vi "Hardware-DiffIO-Host.vi"() -> ()   [LabVIEW 2016]
uses:
  <vilib>/Powertrain Controls/Device Drivers/DCM/Diff IO/RT/Setup.ctl
  <vilib>/Powertrain Controls/Device Drivers/DCM/Diff IO/FPGA/Mode.ctl
  <vilib>/Powertrain Controls/Device Drivers/DCM/Diff IO/RT/Angle Control.ctl
  <vilib>/Powertrain Controls/Device Drivers/DCM/Diff IO/RT/Results.ctl
  Shared/Typedefs/DiffIO-PWM-Settings.ctl
  Shared/Typedefs/DiffIO-PWM-Settings-Array.ctl
  <vilib>/Powertrain Controls/Device Drivers/DCM/Diff IO/FPGA/DCM - FPGA - Diff IO.lvlib
  Shared/DSI-Shared.lvlib
  <vilib>/Powertrain Controls/Device Drivers/DCM/Diff IO/RT/DCM - RT - Diff IO.lvlib
panel:
  in  "_Hidden":enum32{"Page 1"}(tab)
  in  "Setup":T1[](array[typedef])=[{"Mode"=enum."Off", "Capture Start [DBTDC]"=0.0, "Capture End [DBTDC]"=0.0, "Polarity"=FALSE, "Frequency [Hz]"=0.0, "Duty Cycle [%]"=0.0, "TDC Offset [CAD]"=0.0, "Window Start [DBTDC]"=0.0, "Window End [DBTDC]"=0.0, "Angles"=[{"Enable"=FALSE, "Location [DBTDC]"=0.0, "Duration [s]"=0.0}, {"Enable"=FALSE, "Location [DBTDC]"=0.0, "Duration [s]"=0.0}, {"Enable"=FALSE, "Location [DBTDC]"=0.0, "Duration [s]"=0.0}, {"Enable"=FALSE, "Location [DBTDC]"=0.0, "Duration [s]"=0.0}], "Skip Fire"=FALSE, "Skip Fire Index"=0}, {"Mode"=enum."Off", "Capture Start [DBTDC]"=0.0, "Capture End [DBTDC]"=0.0, "Polarity"=FALSE, "Frequency [Hz]"=0.0, "Duty Cycle [%]"=0.0, "TDC Offset [CAD]"=0.0, "Window Start [DBTDC]"=0.0, "Window End [DBTDC]"=0.0, "Angles"=[{"Enable"=FALSE, "Location [DBTDC]"=0.0, "Duration [s]"=0.0}, {"Enable"=FALSE, "Location [DBTDC]"=0.0, "Duration [s]"=0.0}, {"Enable"=FALSE, "Location [DBTDC]"=0.0, "Duration [s]"=0.0}, {"Enable"=FALSE, "Location [DBTDC]"=0.0, "Duration [s]"=0.0}], "Skip Fire"=FALSE, "Skip Fire Index"=0}, {"Mode"=enum."Off", "Capture Start [DBTDC]"=0.0, "Capture End [DBTDC]"=0.0, "Polarity"=FALSE, "Frequency [Hz]"=0.0, "Duty Cycle [%]"=0.0, "TDC Offset [CAD]"=0.0, "Window Start [DBTDC]"=0.0, "Window End [DBTDC]"=0.0, "Angles"=[{"Enable"=FALSE, "Location [DBTDC]"=0.0, "Duration [s]"=0.0}, {"Enable"=FALSE, "Location [DBTDC]"=0.0, "Duration [s]"=0.0}, {"Enable"=FALSE, "Location [DBTDC]"=0.0, "Duration [s]"=0.0}, {"Enable"=FALSE, "Location [DBTDC]"=0.0, "Duration [s]"=0.0}], "Skip Fire"=FALSE, "Skip Fire Index"=0}, {"Mode"=enum."Off", "Capture Start [DBTDC]"=0.0, "Capture End [DBTDC]"=0.0, "Polarity"=FALSE, "Frequency [Hz]"=0.0, "Duty Cycle [%]"=0.0, "TDC Offset [CAD]"=0.0, "Window Start [DBTDC]"=0.0, "Window End [DBTDC]"=0.0, "Angles"=[{"Enable"=FALSE, "Location [DBTDC]"=0.0, "Duration [s]"=0.0}, {"Enable"=FALSE, "Location [DBTDC]"=0.0, "Duration [s]"=0.0}, {"Enable"=FALSE, "Location [DBTDC]"=0.0, "Duration [s]"=0.0}, {"Enable"=FALSE, "Location [DBTDC]"=0.0, "Duration [s]"=0.0}], "Skip Fire"=FALSE, "Skip Fire Index"=0}, {"Mode"=enum."Off", "Capture Start [DBTDC]"=0.0, "Capture End [DBTDC]"=0.0, "Polarity"=FALSE, "Frequency [Hz]"=0.0, "Duty Cycle [%]"=0.0, "TDC Offset [CAD]"=0.0, "Window Start [DBTDC]"=0.0, "Window End [DBTDC]"=0.0, "Angles"=[{"Enable"=FALSE, "Location [DBTDC]"=0.0, "Duration [s]"=0.0}, {"Enable"=FALSE, "Location [DBTDC]"=0.0, "Duration [s]"=0.0}, {"Enable"=FALSE, "Location [DBTDC]"=0.0, "Duration [s]"=0.0}, {"Enable"=FALSE, "Location [DBTDC]"=0.0, "Duration [s]"=0.0}], "Skip Fire"=FALSE, "Skip Fire Index"=0}, {"Mode"=enum."Off", "Capture Start [DBTDC]"=0.0, "Capture End [DBTDC]"=0.0, "Polarity"=FALSE, "Frequency [Hz]"=0.0, "Duty Cycle [%]"=0.0, "TDC Offset [CAD]"=0.0, "Window Start [DBTDC]"=0.0, "Window End [DBTDC]"=0.0, "Angles"=[{"Enable"=FALSE, "Location [DBTDC]"=0.0, "Duration [s]"=0.0}, {"Enable"=FALSE, "Location [DBTDC]"=0.0, "Duration [s]"=0.0}, {"Enable"=FALSE, "Location [DBTDC]"=0.0, "Duration [s]"=0.0}, {"Enable"=FALSE, "Location [DBTDC]"=0.0, "Duration [s]"=0.0}], "Skip Fire"=FALSE, "Skip Fire Index"=0}, {"Mode"=enum."Off", "Capture Start [DBTDC]"=0.0, "Capture End [DBTDC]"=0.0, "Polarity"=FALSE, "Frequency [Hz]"=0.0, "Duty Cycle [%]"=0.0, "TDC Offset [CAD]"=0.0, "Window Start [DBTDC]"=0.0, "Window End [DBTDC]"=0.0, "Angles"=[{"Enable"=FALSE, "Location [DBTDC]"=0.0, "Duration [s]"=0.0}, {"Enable"=FALSE, "Location [DBTDC]"=0.0, "Duration [s]"=0.0}, {"Enable"=FALSE, "Location [DBTDC]"=0.0, "Duration [s]"=0.0}, {"Enable"=FALSE, "Location [DBTDC]"=0.0, "Duration [s]"=0.0}], "Skip Fire"=FALSE, "Skip Fire Index"=0}, {"Mode"=enum."Off", "Capture Start [DBTDC]"=0.0, "Capture End [DBTDC]"=0.0, "Polarity"=FALSE, "Frequency [Hz]"=0.0, "Duty Cycle [%]"=0.0, "TDC Offset [CAD]"=0.0, "Window Start [DBTDC]"=0.0, "Window End [DBTDC]"=0.0, "Angles"=[{"Enable"=FALSE, "Location [DBTDC]"=0.0, "Duration [s]"=0.0}, {"Enable"=FALSE, "Location [DBTDC]"=0.0, "Duration [s]"=0.0}, {"Enable"=FALSE, "Location [DBTDC]"=0.0, "Duration [s]"=0.0}, {"Enable"=FALSE, "Location [DBTDC]"=0.0, "Duration [s]"=0.0}], "Skip Fire"=FALSE, "Skip Fire Index"=0}] {"Skip Fire Index" max=7; "Angles"."Duration [s]" format="%#_3p"; "Frequency [Hz]" format="%#_3p"}
  in  "_Refresh":bool
  in  "AdaptMode":u32
  in  "ChannelNames":string
  out "State":u8
  out "Results":T4[](array[typedef]) {"Duty Cycle [%]" format="%#_3g"; "Frequency [Hz]" format="%#_3p"}
  in  "PWMSettings":T5=[{"PWM-TimingMode"=enum."Frequency", "PWM-Frequency"=0.0, "PWM-Period"=0.0, "PWM-ControlMode"=enum."Duty Cycle", "PWM-DutyCycle"=0.0, "PWM-PulseWidth"=0.0}, {"PWM-TimingMode"=enum."Frequency", "PWM-Frequency"=0.0, "PWM-Period"=0.0, "PWM-ControlMode"=enum."Duty Cycle", "PWM-DutyCycle"=0.0, "PWM-PulseWidth"=0.0}, {"PWM-TimingMode"=enum."Frequency", "PWM-Frequency"=0.0, "PWM-Period"=0.0, "PWM-ControlMode"=enum."Duty Cycle", "PWM-DutyCycle"=0.0, "PWM-PulseWidth"=0.0}, {"PWM-TimingMode"=enum."Frequency", "PWM-Frequency"=0.0, "PWM-Period"=0.0, "PWM-ControlMode"=enum."Duty Cycle", "PWM-DutyCycle"=0.0, "PWM-PulseWidth"=0.0}, {"PWM-TimingMode"=enum."Frequency", "PWM-Frequency"=0.0, "PWM-Period"=0.0, "PWM-ControlMode"=enum."Duty Cycle", "PWM-DutyCycle"=0.0, "PWM-PulseWidth"=0.0}, {"PWM-TimingMode"=enum."Frequency", "PWM-Frequency"=0.0, "PWM-Period"=0.0, "PWM-ControlMode"=enum."Duty Cycle", "PWM-DutyCycle"=0.0, "PWM-PulseWidth"=0.0}, {"PWM-TimingMode"=enum."Frequency", "PWM-Frequency"=0.0, "PWM-Period"=0.0, "PWM-ControlMode"=enum."Duty Cycle", "PWM-DutyCycle"=0.0, "PWM-PulseWidth"=0.0}, {"PWM-TimingMode"=enum."Frequency", "PWM-Frequency"=0.0, "PWM-Period"=0.0, "PWM-ControlMode"=enum."Duty Cycle", "PWM-DutyCycle"=0.0, "PWM-PulseWidth"=0.0}] caption="Advanced PWM Settings" {"PWM-Period" format="%#_2p"; "PWM-PulseWidth" format="%#_2p"; "PWM-DutyCycle" format="%#_2p"; "PWM-Frequency" format="%#_2p"}
  in  "Filters":sgl[](array[numeric]) caption="Digital Filter" format="%#.2p"
  in  "_Filter":sgl caption="Digital Filter [s]" format="%#_4p"
  in  "_PWM Settings Element":T6 caption="Advanced PWM Settings" {"PWM-Period" format="%#_2p"; "PWM-PulseWidth" format="%#_2p"; "PWM-DutyCycle" format="%#_2p"; "PWM-Frequency" format="%#_2p"}
  in  "_Setup Tab":enum32{"Page 1"}(tab)
  out "_ResultsElement":T4 caption="Channel Results" {"Duty Cycle [%]" format="%#_3g"; "Frequency [Hz]" format="%#_3p"}
  in  "_SetupElement":T1={"Mode"=enum."Off", "Capture Start [DBTDC]"=0.0, "Capture End [DBTDC]"=0.0, "Polarity"=FALSE, "Frequency [Hz]"=0.0, "Duty Cycle [%]"=0.0, "TDC Offset [CAD]"=0.0, "Window Start [DBTDC]"=0.0, "Window End [DBTDC]"=0.0, "Angles"=[{"Enable"=FALSE, "Location [DBTDC]"=0.0, "Duration [s]"=0.0}, {"Enable"=FALSE, "Location [DBTDC]"=0.0, "Duration [s]"=0.0}, {"Enable"=FALSE, "Location [DBTDC]"=0.0, "Duration [s]"=0.0}, {"Enable"=FALSE, "Location [DBTDC]"=0.0, "Duration [s]"=0.0}], "Skip Fire"=FALSE, "Skip Fire Index"=0} caption="Command Setup" {"Skip Fire Index" max=7; "Angles"."Duration [s]" format="%#_3p"; "Frequency [Hz]" format="%#_3p"}
  in  "_AdaptMode":bool caption="Adapt Mode"
  in  "_Channel Name":string caption="Name"
  in  "_DiffIO Channels":i32[](listbox) caption="Differential Digital I/O Channel Summary"
  # "Differential Digital I/O Setup & Control"
  # "Channel Settings"
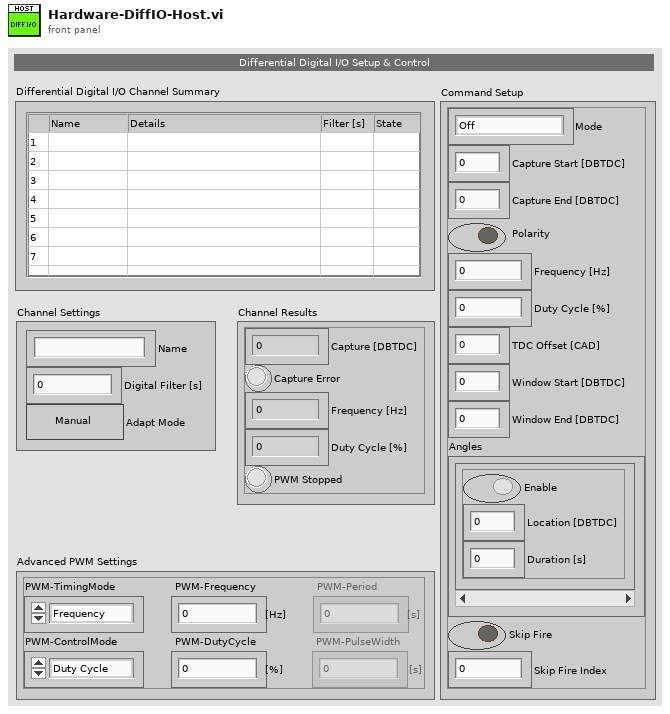
[diagram p1: front panel]
types:
  T1 = typedef "DCM - RT - Diff IO.lvlib/Setup.ctl" = cluster{"Mode":T2, "Capture Start [DBTDC]":sgl, "Capture End [DBTDC]":sgl, "Polarity":bool, "Frequency [Hz]":sgl, "Duty Cycle [%]":sgl, "TDC Offset [CAD]":sgl, "Window Start [DBTDC]":sgl, "Window End [DBTDC]":sgl, "Angles":T3[], "Skip Fire":bool, "Skip Fire Index":u8}
  T2 = typedef "DCM - FPGA - Diff IO.lvlib/Mode.ctl" = enum8{"Off", "Input", "Pulse Width Modulation", "Engine Position Tracking", "Serial Out 1", "Serial Out 2"}
  T3 = typedef "DCM - RT - Diff IO.lvlib/Angle Control.ctl" = cluster{"Enable":bool, "Location [DBTDC]":sgl, "Duration [s]":sgl}
  T4 = typedef "DCM - RT - Diff IO.lvlib/Results.ctl" = cluster{"Capture [DBTDC]":sgl, "Capture Error":bool, "Frequency [Hz]":sgl, "Duty Cycle [%]":sgl, "PWM Stopped":bool}
  T5 = typedef "DSI-Shared.lvlib/DiffIO-PWM-Settings-Array.ctl" = T6[]
  T6 = typedef "DSI-Shared.lvlib/DiffIO-PWM-Settings.ctl" = cluster{"PWM-TimingMode":enum32{"Frequency", "Period"}, "PWM-Frequency":sgl, "PWM-Period":sgl, "PWM-ControlMode":enum32{"Duty Cycle", "Pulsewidth"}, "PWM-DutyCycle":sgl, "PWM-PulseWidth":sgl}
  T7 = enum8{"Enabled", "Disabled", "Disabled and Grayed Out"}
  T8 = enum32{"Invalid", "Standard", "Closed", "Hidden", "Minimized", "Maximized"}
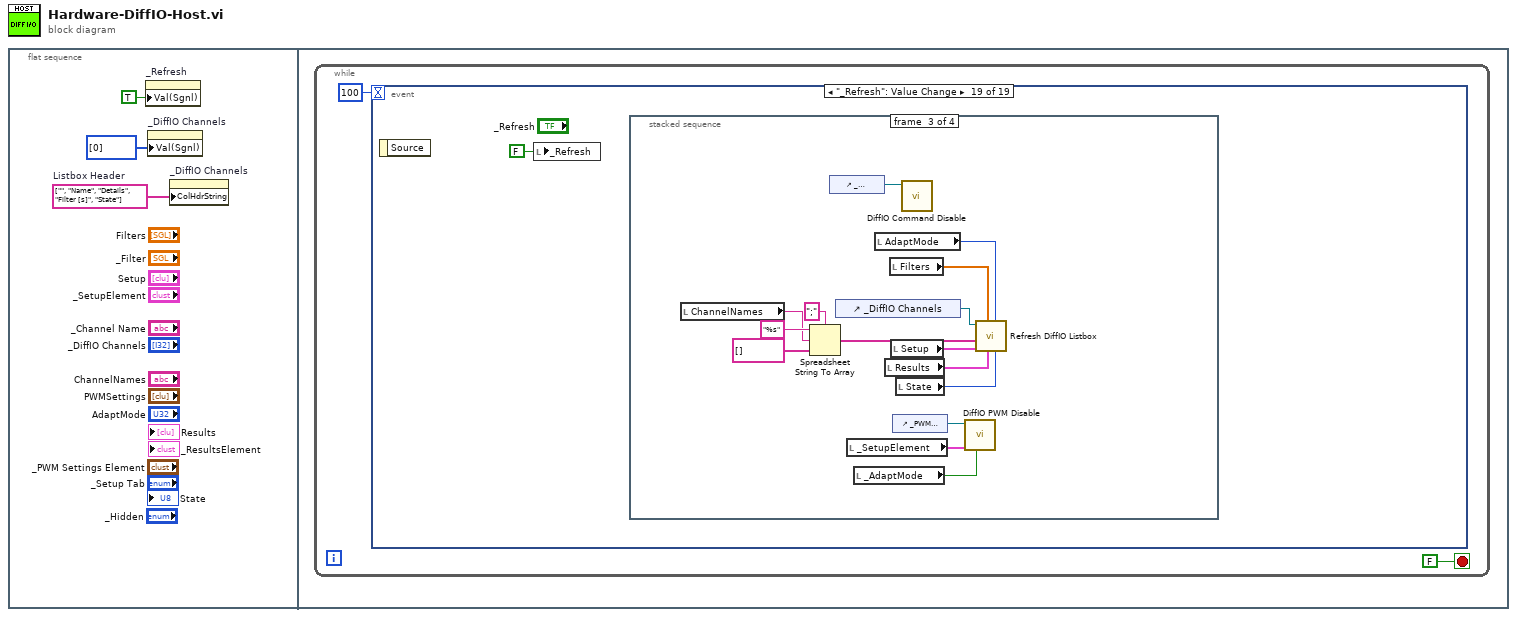
[diagram p0: block diagram]
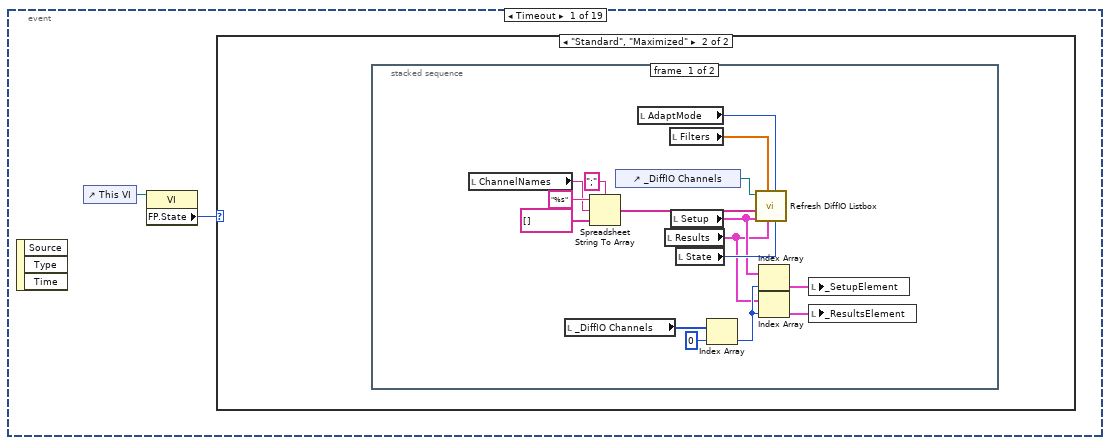
[diagram p2: hidden frame]
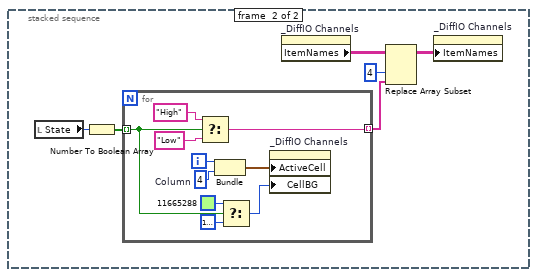
[diagram p4: hidden frame]
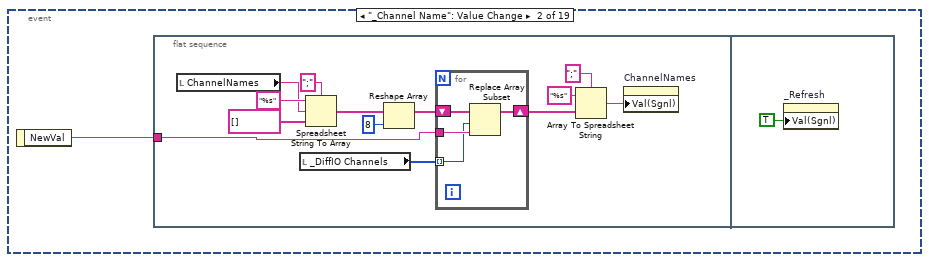
[diagram p5: hidden frame]
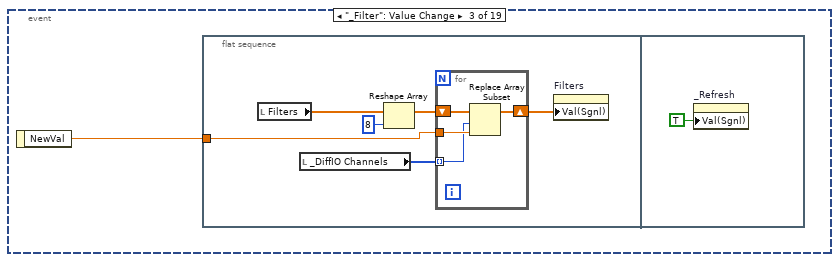
[diagram p6: hidden frame]
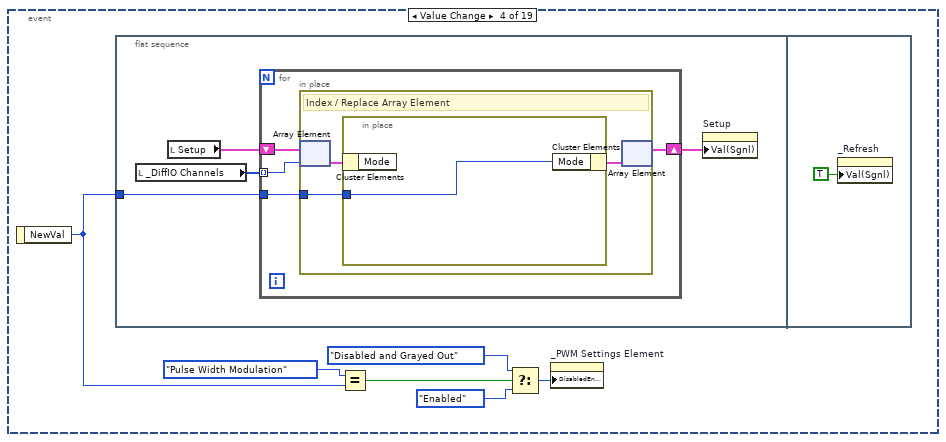
[diagram p7: hidden frame]
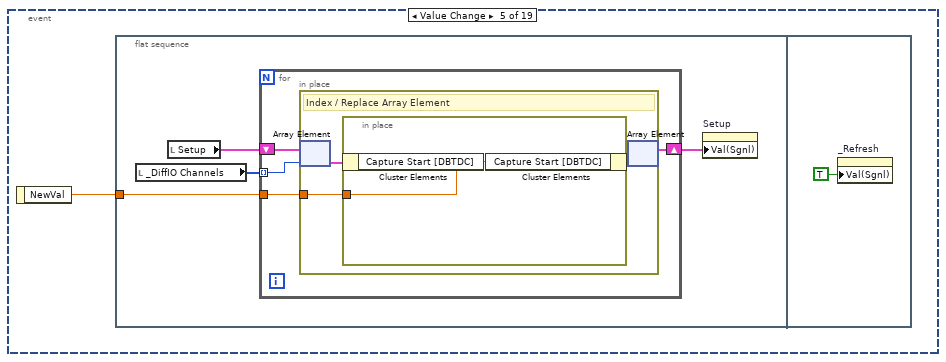
[diagram p8: hidden frame]
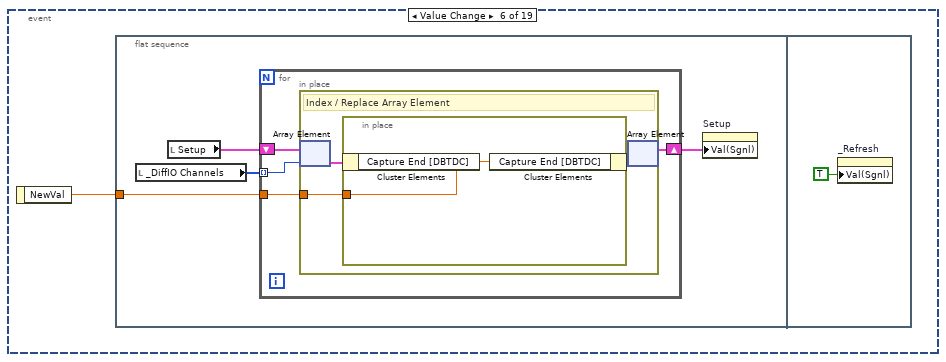
[diagram p9: hidden frame]
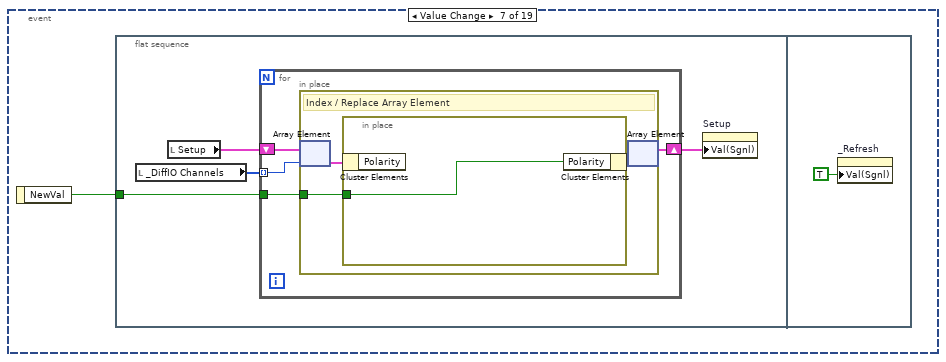
[diagram p10: hidden frame]
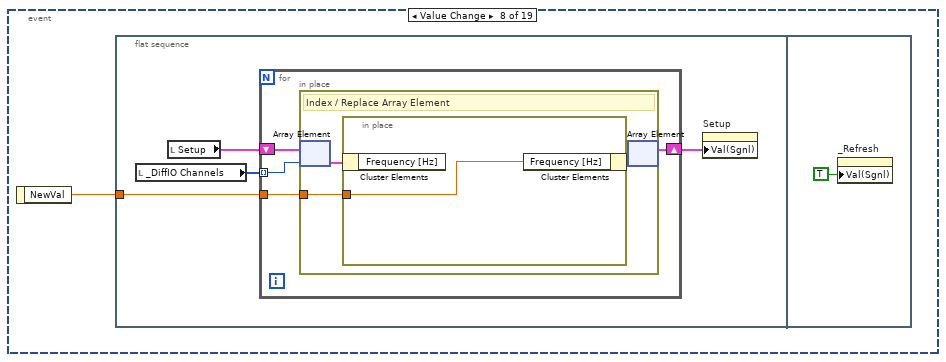
[diagram p11: hidden frame]
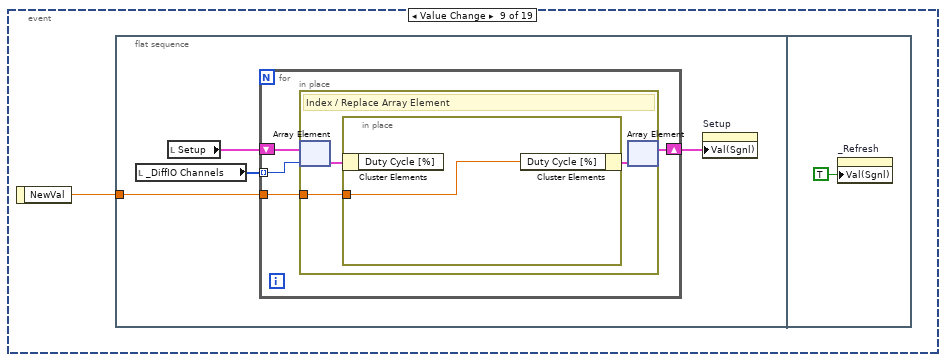
[diagram p12: hidden frame]
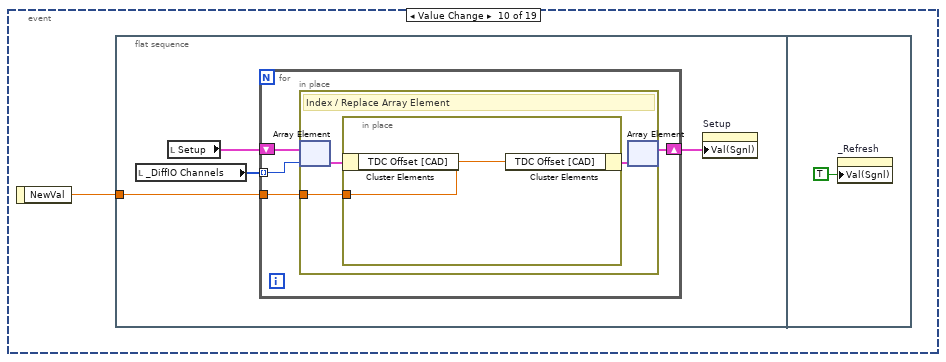
[diagram p13: hidden frame]
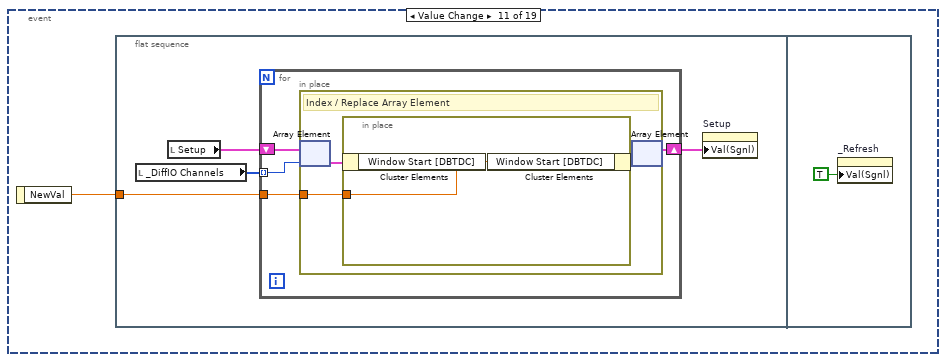
[diagram p14: hidden frame]
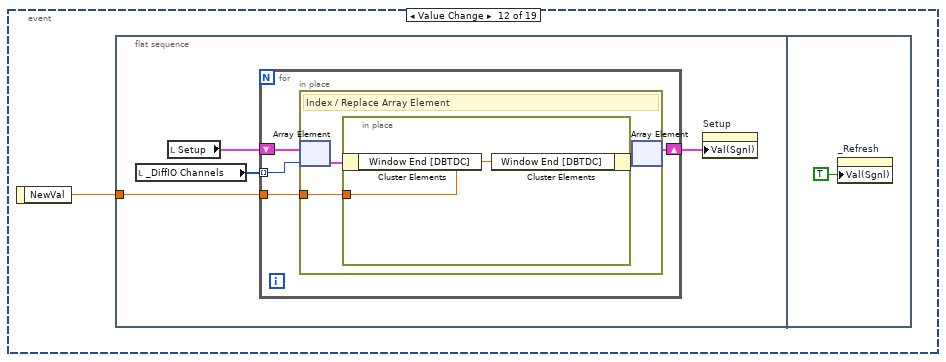
[diagram p15: hidden frame]
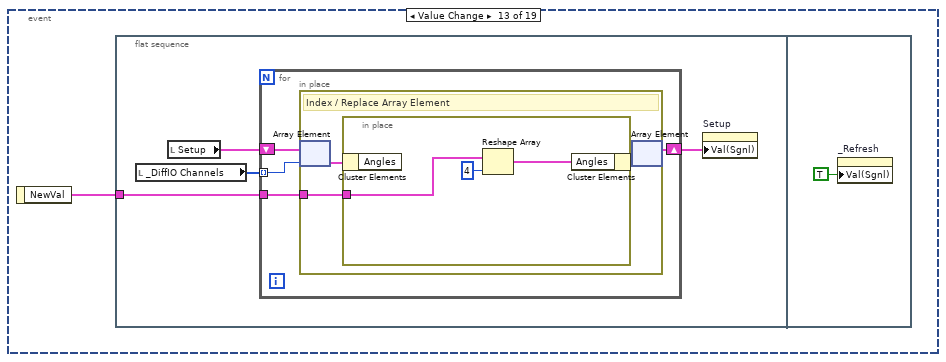
[diagram p16: hidden frame]
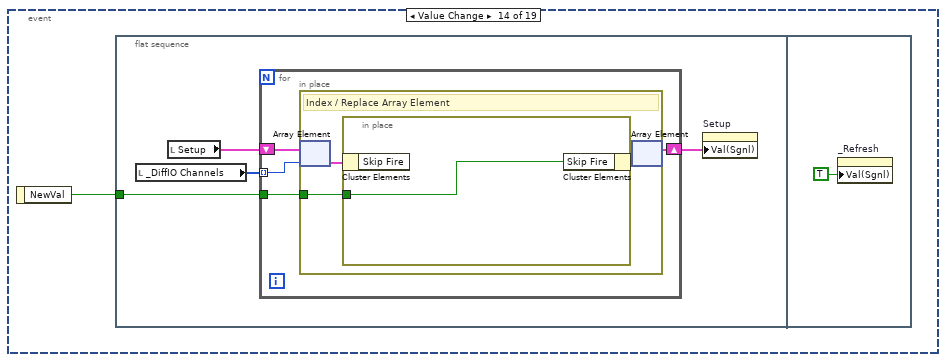
[diagram p17: hidden frame]
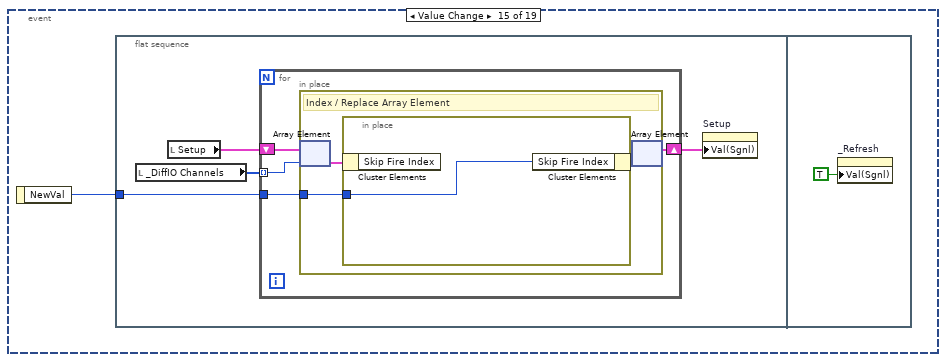
[diagram p18: hidden frame]
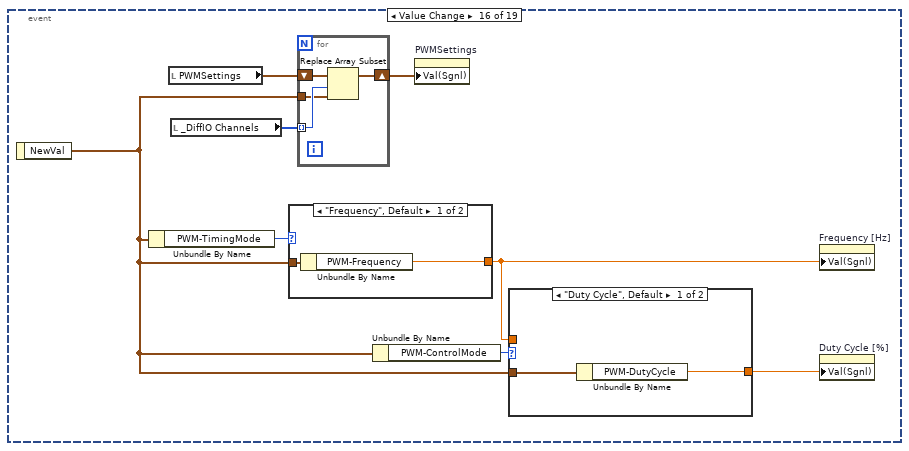
[diagram p19: hidden frame]
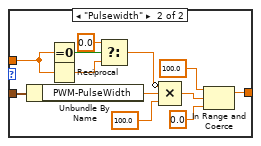
[diagram p20: hidden frame]
diagram:
  n1 = flat-sequence "Initialization code" {
    frame #0 {
      w3 = string[] ["", "Name", "Details", "Filter [s]", "State"]  # Listbox Header
      n2 = property on="_Refresh" class="Bool (strict)"("Val(Sgnl)"=TRUE ("Value (Signaling)")) -> ()  [unwired: 2 in, 2 out]
      n3 = property on="_DiffIO Channels" class="MCListbox (strict)"("Val(Sgnl)"=i32[] [0] ("Value (Signaling)")) -> ()  [unwired: 2 in, 2 out]
      n4 = property on="_DiffIO Channels" class="MCListbox (strict)"("ColHdrString"=w3) -> ()  [unwired: 2 in, 2 out]
    }
    frame #1 {
      n5 = while {
        stop <- FALSE stop-if-true
        n6 = event shown="[18] \"_Refresh\": Value Change" {
          selector: _ -> [_ _ _ _ _ _ _ _ _ _ _ _ _ _ _ _ _ _ _]
          dyn-events: _ -> [_ _ _ _ _ _ _ _ _ _ _ _ _ _ _ _ _ _ _]
          timeout: 100 -> [_ _ _ _ _ _ _ _ _ _ _ _ _ _ _ _ _ _ _]
          event Timeout {
            n7 = event-data() -> ()  [unwired: 4 out]
            n8 = control-ref of="This VI"() -> (w7:refnum<vi>)
            n9 = property class="VI"(reference=w7) -> ("FP.State"=w6:T8)  [unwired: 1 in, 2 out]
            n10 = case shown="\"Standard\", \"Maximized\"" w6 {
              frame "Invalid", Default {
              }
              frame "Standard", "Maximized" {
                n11 = stacked-sequence {
                  frame #0 {
                    n12 = local read "ChannelNames"() -> (w17:string)
                    n13 = local read "_DiffIO Channels"() -> (w22:i32[])
                    n14 = Spreadsheet String To Array(delimiter (Tab)=";", format string="%s", spreadsheet string=w17, array type (2D Dbl)=string[] []) -> (array=w16:string[])
                    n15 = control-ref of="_DiffIO Channels"() -> (w13:refnum<vi>)
                    n16 = local read "AdaptMode"() -> (w23:u32)
                    n17 = local read "Results"() -> (w8:T4[])
                    n18 = local read "Filters"() -> (w12:sgl[])
                    n19 = local read "Setup"() -> (w9:T1[])
                    n20 = local read "State"() -> (w14:u8)
                    n21 = Index Array(array=w22, index=0) -> (element=w10:i32)
                    n22 = call "Refresh DiffIO Listbox.vi"("_DiffIOState"=w14, "AdaptMode"=w23, "Results"=w8, "DigitalFilter"=w12, "Command"=w9, "Names"=w16, "_DiffIO Channels"=w13) -> ()  [unwired: 5 in]
                    n23 = Index Array(array=w9, index=w10) -> (element=w11:T1)
                    n24 = Index Array(array=w8, index=w10) -> (element=w20:T4)
                    n25 = local write "_SetupElement"(w11) -> ()
                    n26 = local write "_ResultsElement"(w20) -> ()
                  }
                  frame #1 {
                    n27 = local read "State"() -> (w27:u8)
                    n28 = Number To Boolean Array(number=w27) -> (Boolean array=w28:bool[])
                    n29 = for {
                      tunnel: w28 -> [w31] mode=indexing
                      tunnel: [w30] -> w25 mode=indexing
                      i -> [w38]
                      w39 = 4  # Column
                      n30 = Select(t="High" ("format string"), s=w31, f="Low" ("format string")) -> (s? t:f=w30:string)
                      n31 = Bundle(w38, "Column"=w39) -> (w37:cluster{i32, "Column":i32})  [unwired: 1 in]
                      n32 = Select(t=u32 11665288, s=w31, f=u32 16777226) -> (s? t:f=w34:u32)
                      n33 = property on="_DiffIO Channels" class="MCListbox (strict)"("ActiveCell"=w37, "CellBG"=w34) -> ()  [unwired: 2 in, 2 out]
                    }
                    n34 = property on="_DiffIO Channels" class="MCListbox (strict)"() -> ("ItemNames"=w26:string[][])  [unwired: 2 in, 2 out]
                    n35 = Replace Array Subset(array=w26, new element=w25, index (col)=4 ("disabled index (col)")) -> (w24:string[][])  [unwired: 1 in]
                    n36 = property on="_DiffIO Channels" class="MCListbox (strict)"("ItemNames"=w24) -> ()  [unwired: 2 in, 2 out]
                  }
                }
              }
            }
          }
          event "_Channel Name": Value Change {
            n37 = event-data() -> ("NewVal"=w40:string)  [unwired: 1 out]
            n38 = flat-sequence {
              tunnel: w40 -> [w42]
              frame #0 {
                n39 = local read "ChannelNames"() -> (w51:string)
                n40 = local read "_DiffIO Channels"() -> (w41:i32[])
                n41 = Spreadsheet String To Array(delimiter (Tab)=";", format string="%s", spreadsheet string=w51, array type (2D Dbl)=string[] []) -> (array=w49:string[])
                n42 = Reshape Array(w49, 8 ("dimension size")) -> (w44:string[])
                n43 = for {
                  tunnel: w42 -> [w55]
                  shift-right: [w57] -> w48
                  shift-left: w44 -> [w56]
                  tunnel: w41 -> [w54] mode=indexing
                  n44 = Replace Array Subset(array=w56, new element=w55, index=w54) -> (w57:string[])
                }
                n45 = Array To Spreadsheet String(delimiter (Tab)=";", array=w48, 3:"%s" ("format string")) -> (spreadsheet string=w45:string)
                n46 = property on="ChannelNames" class="Str"("Val(Sgnl)"=w45) -> ()  [unwired: 2 in, 2 out]
              }
              frame #1 {
                n47 = property on="_Refresh" class="Bool (strict)"("Val(Sgnl)"=TRUE ("Value (Signaling)")) -> ()  [unwired: 2 in, 2 out]
              }
            }
          }
          event "_Filter": Value Change {
            n48 = event-data() -> ("NewVal"=w59:sgl)  [unwired: 1 out]
            n49 = flat-sequence {
              tunnel: w59 -> [w63]
              frame #0 {
                n50 = local read "Filters"() -> (w61:sgl[])
                n51 = local read "_DiffIO Channels"() -> (w62:i32[])
                n52 = Reshape Array(w61, 8 ("dimension size")) -> (w65:sgl[])
                n53 = for {
                  tunnel: w63 -> [w67]
                  shift-right: [w69] -> w60
                  shift-left: w65 -> [w68]
                  tunnel: w62 -> [w66] mode=indexing
                  n54 = Replace Array Subset(array=w68, new element=w67, index=w66) -> (w69:sgl[])
                }
                n55 = property on="Filters" class="Arr (strict)"("Val(Sgnl)"=w60) -> ()  [unwired: 2 in, 2 out]
              }
              frame #1 {
                n56 = property on="_Refresh" class="Bool (strict)"("Val(Sgnl)"=TRUE ("Value (Signaling)")) -> ()  [unwired: 2 in, 2 out]
              }
            }
          }
          event Value Change {
            n57 = event-data() -> ("NewVal"=w71:T2)  [unwired: 1 out]
            n58 = flat-sequence {
              tunnel: w71 -> [w79]
              frame #0 {
                n59 = local read "_DiffIO Channels"() -> (w80:i32[])
                n60 = local read "Setup"() -> (w78:T1[])
                n61 = for {
                  tunnel: w80 -> [w83] mode=indexing
                  shift-right: [w82] -> w77
                  shift-left: w78 -> [w84]
                  tunnel: w79 -> [w81]
                  n62 = in-place {
                    in-place-border: w81 -> [w85]
                    # "Index / Replace Array Element"
                    n63 = in-place-array #1(w84, w83) -> (w87:T1)
                    n64 = in-place {
                      in-place-border: w85 -> [w88]
                      n65 = in-place-cluster #2(w87) -> ()  [unwired: 1 out]
                      n66 = in-place-cluster #2("Mode"=w88) -> (w86:T1)
                    }
                    n67 = in-place-array #1(w86) -> (w82:T1[])  [unwired: 1 out]
                  }
                }
                n68 = property on="Setup" class="Arr (strict)"("Val(Sgnl)"=w77) -> ()  [unwired: 2 in, 2 out]
              }
              frame #1 {
                n69 = property on="_Refresh" class="Bool (strict)"("Val(Sgnl)"=TRUE ("Value (Signaling)")) -> ()  [unwired: 2 in, 2 out]
              }
            }
            n70 = Equal?(x=Mode."Pulse Width Modulation" ("Mode"), y=w71) -> (x = y?=w73:bool)
            n71 = Select(t=T7."Disabled and Grayed Out" ("Disabled"), s=w73, f=T7."Enabled" ("Disabled")) -> (s? t:f=w72:T7)
            n72 = property on="_PWM Settings Element" class="Clust (strict)"("DisabledEnum"=w72) -> ()  [unwired: 2 in, 2 out]
          }
          event Value Change {
            n73 = event-data() -> ("NewVal"=w90:sgl)  [unwired: 1 out]
            n74 = flat-sequence {
              tunnel: w90 -> [w93]
              frame #0 {
                n75 = local read "_DiffIO Channels"() -> (w94:i32[])
                n76 = local read "Setup"() -> (w92:T1[])
                n77 = for {
                  tunnel: w94 -> [w97] mode=indexing
                  shift-right: [w96] -> w91
                  shift-left: w92 -> [w98]
                  tunnel: w93 -> [w95]
                  n78 = in-place {
                    in-place-border: w95 -> [w99]
                    # "Index / Replace Array Element"
                    n79 = in-place-array #3(w98, w97) -> (w101:T1)
                    n80 = in-place {
                      in-place-border: w99 -> [w102]
                      n81 = in-place-cluster #4(w101) -> ()  [unwired: 1 out]
                      n82 = in-place-cluster #4("Capture Start [DBTDC]"=w102) -> (w100:T1)
                    }
                    n83 = in-place-array #3(w100) -> (w96:T1[])  [unwired: 1 out]
                  }
                }
                n84 = property on="Setup" class="Arr (strict)"("Val(Sgnl)"=w91) -> ()  [unwired: 2 in, 2 out]
              }
              frame #1 {
                n85 = property on="_Refresh" class="Bool (strict)"("Val(Sgnl)"=TRUE ("Value (Signaling)")) -> ()  [unwired: 2 in, 2 out]
              }
            }
          }
          event Value Change {
            n86 = event-data() -> ("NewVal"=w104:sgl)  [unwired: 1 out]
            n87 = flat-sequence {
              tunnel: w104 -> [w107]
              frame #0 {
                n88 = local read "_DiffIO Channels"() -> (w108:i32[])
                n89 = local read "Setup"() -> (w106:T1[])
                n90 = for {
                  tunnel: w108 -> [w111] mode=indexing
                  shift-right: [w110] -> w105
                  shift-left: w106 -> [w112]
                  tunnel: w107 -> [w109]
                  n91 = in-place {
                    in-place-border: w109 -> [w113]
                    # "Index / Replace Array Element"
                    n92 = in-place-array #5(w112, w111) -> (w115:T1)
                    n93 = in-place {
                      in-place-border: w113 -> [w116]
                      n94 = in-place-cluster #6(w115) -> ()  [unwired: 1 out]
                      n95 = in-place-cluster #6("Capture End [DBTDC]"=w116) -> (w114:T1)
                    }
                    n96 = in-place-array #5(w114) -> (w110:T1[])  [unwired: 1 out]
                  }
                }
                n97 = property on="Setup" class="Arr (strict)"("Val(Sgnl)"=w105) -> ()  [unwired: 2 in, 2 out]
              }
              frame #1 {
                n98 = property on="_Refresh" class="Bool (strict)"("Val(Sgnl)"=TRUE ("Value (Signaling)")) -> ()  [unwired: 2 in, 2 out]
              }
            }
          }
          event Value Change {
            n99 = event-data() -> ("NewVal"=w118:bool)  [unwired: 1 out]
            n100 = flat-sequence {
              tunnel: w118 -> [w121]
              frame #0 {
                n101 = local read "_DiffIO Channels"() -> (w122:i32[])
                n102 = local read "Setup"() -> (w120:T1[])
                n103 = for {
                  tunnel: w122 -> [w125] mode=indexing
                  shift-right: [w124] -> w119
                  shift-left: w120 -> [w126]
                  tunnel: w121 -> [w123]
                  n104 = in-place {
                    in-place-border: w123 -> [w127]
                    # "Index / Replace Array Element"
                    n105 = in-place-array #7(w126, w125) -> (w129:T1)
                    n106 = in-place {
                      in-place-border: w127 -> [w130]
                      n107 = in-place-cluster #8(w129) -> ()  [unwired: 1 out]
                      n108 = in-place-cluster #8("Polarity"=w130) -> (w128:T1)
                    }
                    n109 = in-place-array #7(w128) -> (w124:T1[])  [unwired: 1 out]
                  }
                }
                n110 = property on="Setup" class="Arr (strict)"("Val(Sgnl)"=w119) -> ()  [unwired: 2 in, 2 out]
              }
              frame #1 {
                n111 = property on="_Refresh" class="Bool (strict)"("Val(Sgnl)"=TRUE ("Value (Signaling)")) -> ()  [unwired: 2 in, 2 out]
              }
            }
          }
          event Value Change {
            n112 = event-data() -> ("NewVal"=w132:sgl)  [unwired: 1 out]
            n113 = flat-sequence {
              tunnel: w132 -> [w135]
              frame #0 {
                n114 = local read "_DiffIO Channels"() -> (w136:i32[])
                n115 = local read "Setup"() -> (w134:T1[])
                n116 = for {
                  tunnel: w136 -> [w139] mode=indexing
                  shift-right: [w138] -> w133
                  shift-left: w134 -> [w140]
                  tunnel: w135 -> [w137]
                  n117 = in-place {
                    in-place-border: w137 -> [w141]
                    # "Index / Replace Array Element"
                    n118 = in-place-array #9(w140, w139) -> (w143:T1)
                    n119 = in-place {
                      in-place-border: w141 -> [w144]
                      n120 = in-place-cluster #10(w143) -> ()  [unwired: 1 out]
                      n121 = in-place-cluster #10("Frequency [Hz]"=w144) -> (w142:T1)
                    }
                    n122 = in-place-array #9(w142) -> (w138:T1[])  [unwired: 1 out]
                  }
                }
                n123 = property on="Setup" class="Arr (strict)"("Val(Sgnl)"=w133) -> ()  [unwired: 2 in, 2 out]
              }
              frame #1 {
                n124 = property on="_Refresh" class="Bool (strict)"("Val(Sgnl)"=TRUE ("Value (Signaling)")) -> ()  [unwired: 2 in, 2 out]
              }
            }
          }
          event Value Change {
            n125 = event-data() -> ("NewVal"=w146:sgl)  [unwired: 1 out]
            n126 = flat-sequence {
              tunnel: w146 -> [w149]
              frame #0 {
                n127 = local read "_DiffIO Channels"() -> (w150:i32[])
                n128 = local read "Setup"() -> (w148:T1[])
                n129 = for {
                  tunnel: w150 -> [w153] mode=indexing
                  shift-right: [w152] -> w147
                  shift-left: w148 -> [w154]
                  tunnel: w149 -> [w151]
                  n130 = in-place {
                    in-place-border: w151 -> [w155]
                    # "Index / Replace Array Element"
                    n131 = in-place-array #11(w154, w153) -> (w157:T1)
                    n132 = in-place {
                      in-place-border: w155 -> [w158]
                      n133 = in-place-cluster #12(w157) -> ()  [unwired: 1 out]
                      n134 = in-place-cluster #12("Duty Cycle [%]"=w158) -> (w156:T1)
                    }
                    n135 = in-place-array #11(w156) -> (w152:T1[])  [unwired: 1 out]
                  }
                }
                n136 = property on="Setup" class="Arr (strict)"("Val(Sgnl)"=w147) -> ()  [unwired: 2 in, 2 out]
              }
              frame #1 {
                n137 = property on="_Refresh" class="Bool (strict)"("Val(Sgnl)"=TRUE ("Value (Signaling)")) -> ()  [unwired: 2 in, 2 out]
              }
            }
          }
          event Value Change {
            n138 = event-data() -> ("NewVal"=w160:sgl)  [unwired: 1 out]
            n139 = flat-sequence {
              tunnel: w160 -> [w163]
              frame #0 {
                n140 = local read "_DiffIO Channels"() -> (w164:i32[])
                n141 = local read "Setup"() -> (w162:T1[])
                n142 = for {
                  tunnel: w164 -> [w167] mode=indexing
                  shift-right: [w166] -> w161
                  shift-left: w162 -> [w168]
                  tunnel: w163 -> [w165]
                  n143 = in-place {
                    in-place-border: w165 -> [w169]
                    # "Index / Replace Array Element"
                    n144 = in-place-array #13(w168, w167) -> (w171:T1)
                    n145 = in-place {
                      in-place-border: w169 -> [w172]
                      n146 = in-place-cluster #14(w171) -> ()  [unwired: 1 out]
                      n147 = in-place-cluster #14("TDC Offset [CAD]"=w172) -> (w170:T1)
                    }
                    n148 = in-place-array #13(w170) -> (w166:T1[])  [unwired: 1 out]
                  }
                }
                n149 = property on="Setup" class="Arr (strict)"("Val(Sgnl)"=w161) -> ()  [unwired: 2 in, 2 out]
              }
              frame #1 {
                n150 = property on="_Refresh" class="Bool (strict)"("Val(Sgnl)"=TRUE ("Value (Signaling)")) -> ()  [unwired: 2 in, 2 out]
              }
            }
          }
          event Value Change {
            n151 = event-data() -> ("NewVal"=w174:sgl)  [unwired: 1 out]
            n152 = flat-sequence {
              tunnel: w174 -> [w177]
              frame #0 {
                n153 = local read "_DiffIO Channels"() -> (w178:i32[])
                n154 = local read "Setup"() -> (w176:T1[])
                n155 = for {
                  tunnel: w178 -> [w181] mode=indexing
                  shift-right: [w180] -> w175
                  shift-left: w176 -> [w182]
                  tunnel: w177 -> [w179]
                  n156 = in-place {
                    in-place-border: w179 -> [w183]
                    # "Index / Replace Array Element"
                    n157 = in-place-array #15(w182, w181) -> (w185:T1)
                    n158 = in-place {
                      in-place-border: w183 -> [w186]
                      n159 = in-place-cluster #16(w185) -> ()  [unwired: 1 out]
                      n160 = in-place-cluster #16("Window Start [DBTDC]"=w186) -> (w184:T1)
                    }
                    n161 = in-place-array #15(w184) -> (w180:T1[])  [unwired: 1 out]
                  }
                }
                n162 = property on="Setup" class="Arr (strict)"("Val(Sgnl)"=w175) -> ()  [unwired: 2 in, 2 out]
              }
              frame #1 {
                n163 = property on="_Refresh" class="Bool (strict)"("Val(Sgnl)"=TRUE ("Value (Signaling)")) -> ()  [unwired: 2 in, 2 out]
              }
            }
          }
          event Value Change {
            n164 = event-data() -> ("NewVal"=w188:sgl)  [unwired: 1 out]
            n165 = flat-sequence {
              tunnel: w188 -> [w191]
              frame #0 {
                n166 = local read "_DiffIO Channels"() -> (w192:i32[])
                n167 = local read "Setup"() -> (w190:T1[])
                n168 = for {
                  tunnel: w192 -> [w195] mode=indexing
                  shift-right: [w194] -> w189
                  shift-left: w190 -> [w196]
                  tunnel: w191 -> [w193]
                  n169 = in-place {
                    in-place-border: w193 -> [w197]
                    # "Index / Replace Array Element"
                    n170 = in-place-array #17(w196, w195) -> (w199:T1)
                    n171 = in-place {
                      in-place-border: w197 -> [w200]
                      n172 = in-place-cluster #18(w199) -> ()  [unwired: 1 out]
                      n173 = in-place-cluster #18("Window End [DBTDC]"=w200) -> (w198:T1)
                    }
                    n174 = in-place-array #17(w198) -> (w194:T1[])  [unwired: 1 out]
                  }
                }
                n175 = property on="Setup" class="Arr (strict)"("Val(Sgnl)"=w189) -> ()  [unwired: 2 in, 2 out]
              }
              frame #1 {
                n176 = property on="_Refresh" class="Bool (strict)"("Val(Sgnl)"=TRUE ("Value (Signaling)")) -> ()  [unwired: 2 in, 2 out]
              }
            }
          }
          event Value Change {
            n177 = event-data() -> ("NewVal"=w202:T3[])  [unwired: 1 out]
            n178 = flat-sequence {
              tunnel: w202 -> [w205]
              frame #0 {
                n179 = local read "_DiffIO Channels"() -> (w206:i32[])
                n180 = local read "Setup"() -> (w204:T1[])
                n181 = for {
                  tunnel: w206 -> [w209] mode=indexing
                  shift-right: [w208] -> w203
                  shift-left: w204 -> [w210]
                  tunnel: w205 -> [w207]
                  n182 = in-place {
                    in-place-border: w207 -> [w211]
                    # "Index / Replace Array Element"
                    n183 = in-place-array #19(w210, w209) -> (w213:T1)
                    n184 = in-place {
                      in-place-border: w211 -> [w215]
                      n185 = in-place-cluster #20(w213) -> ()  [unwired: 1 out]
                      n186 = Reshape Array(w215, 4 ("dimension size")) -> (w214:T3[])
                      n187 = in-place-cluster #20("Angles"=w214) -> (w212:T1)
                    }
                    n188 = in-place-array #19(w212) -> (w208:T1[])  [unwired: 1 out]
                  }
                }
                n189 = property on="Setup" class="Arr (strict)"("Val(Sgnl)"=w203) -> ()  [unwired: 2 in, 2 out]
              }
              frame #1 {
                n190 = property on="_Refresh" class="Bool (strict)"("Val(Sgnl)"=TRUE ("Value (Signaling)")) -> ()  [unwired: 2 in, 2 out]
              }
            }
          }
          event Value Change {
            n191 = event-data() -> ("NewVal"=w218:bool)  [unwired: 1 out]
            n192 = flat-sequence {
              tunnel: w218 -> [w221]
              frame #0 {
                n193 = local read "_DiffIO Channels"() -> (w222:i32[])
                n194 = local read "Setup"() -> (w220:T1[])
                n195 = for {
                  tunnel: w222 -> [w225] mode=indexing
                  shift-right: [w224] -> w219
                  shift-left: w220 -> [w226]
                  tunnel: w221 -> [w223]
                  n196 = in-place {
                    in-place-border: w223 -> [w227]
                    # "Index / Replace Array Element"
                    n197 = in-place-array #21(w226, w225) -> (w229:T1)
                    n198 = in-place {
                      in-place-border: w227 -> [w230]
                      n199 = in-place-cluster #22(w229) -> ()  [unwired: 1 out]
                      n200 = in-place-cluster #22("Skip Fire"=w230) -> (w228:T1)
                    }
                    n201 = in-place-array #21(w228) -> (w224:T1[])  [unwired: 1 out]
                  }
                }
                n202 = property on="Setup" class="Arr (strict)"("Val(Sgnl)"=w219) -> ()  [unwired: 2 in, 2 out]
              }
              frame #1 {
                n203 = property on="_Refresh" class="Bool (strict)"("Val(Sgnl)"=TRUE ("Value (Signaling)")) -> ()  [unwired: 2 in, 2 out]
              }
            }
          }
          event Value Change {
            n204 = event-data() -> ("NewVal"=w232:u8)  [unwired: 1 out]
            n205 = flat-sequence {
              tunnel: w232 -> [w235]
              frame #0 {
                n206 = local read "_DiffIO Channels"() -> (w236:i32[])
                n207 = local read "Setup"() -> (w234:T1[])
                n208 = for {
                  tunnel: w236 -> [w239] mode=indexing
                  shift-right: [w238] -> w233
                  shift-left: w234 -> [w240]
                  tunnel: w235 -> [w237]
                  n209 = in-place {
                    in-place-border: w237 -> [w241]
                    # "Index / Replace Array Element"
                    n210 = in-place-array #23(w240, w239) -> (w243:T1)
                    n211 = in-place {
                      in-place-border: w241 -> [w244]
                      n212 = in-place-cluster #24(w243) -> ()  [unwired: 1 out]
                      n213 = in-place-cluster #24("Skip Fire Index"=w244) -> (w242:T1)
                    }
                    n214 = in-place-array #23(w242) -> (w238:T1[])  [unwired: 1 out]
                  }
                }
                n215 = property on="Setup" class="Arr (strict)"("Val(Sgnl)"=w233) -> ()  [unwired: 2 in, 2 out]
              }
              frame #1 {
                n216 = property on="_Refresh" class="Bool (strict)"("Val(Sgnl)"=TRUE ("Value (Signaling)")) -> ()  [unwired: 2 in, 2 out]
              }
            }
          }
          event Value Change {
            n217 = event-data() -> ("NewVal"=w248:T6)  [unwired: 1 out]
            n218 = Unbundle By Name(w248) -> ("PWM-TimingMode"=w252:enum32{"Frequency", "Period"})
            n219 = local read "PWMSettings"() -> (w251:T5)
            n220 = local read "_DiffIO Channels"() -> (w249:i32[])
            n221 = case shown="\"Frequency\", Default" w252 {
              tunnel: w248 -> [w273 w279]
              tunnel: [w272 w276] -> w247
              frame "Frequency", Default {
                n222 = Unbundle By Name(w273) -> ("PWM-Frequency"=w272:sgl)
              }
              frame "Period" {
                n223 = Unbundle By Name(w279) -> ("PWM-Period"=w274:sgl)
                n224 = Equal To 0?(x=w274) -> (x = 0?=w277:bool)
                n225 = Reciprocal(x=w274) -> (1/x=w278:sgl)
                n226 = Select(t=sgl 0.0, s=w277, f=w278) -> (s? t:f=w276:sgl)
              }
            }
            n227 = for {
              shift-right: [w256] -> w250
              shift-left: w251 -> [w255]
              tunnel: w249 -> [w257] mode=indexing
              tunnel: w248 -> [w254]
              n228 = Replace Array Subset(array=w255, new element=w254, index=w257) -> (w256:T5)
            }
            n229 = Unbundle By Name(w248) -> ("PWM-ControlMode"=w253:enum32{"Duty Cycle", "Pulsewidth"})
            n230 = property on="PWMSettings" class="Arr (strict)"("Val(Sgnl)"=w250) -> ()  [unwired: 2 in, 2 out]
            n231 = case shown="\"Duty Cycle\", Default" w253 {
              tunnel: w248 -> [w259 w271]
              tunnel: [w258 w261] -> w246
              tunnel: w247 -> [_ w265]
              frame "Duty Cycle", Default {
                n232 = Unbundle By Name(w259) -> ("PWM-DutyCycle"=w258:sgl)
              }
              frame "Pulsewidth" {
                n233 = Unbundle By Name(w271) -> ("PWM-PulseWidth"=w270:sgl)
                n234 = Equal To 0?(x=w265) -> (x = 0?=w268:bool)
                n235 = Reciprocal(x=w265) -> (1/x=w269:sgl)
                n236 = Select(t=sgl 0.0, s=w268, f=w269) -> (s? t:f=w266:sgl)
                n237 = Compound Arithmetic op=MULTIPLY(invert w266, w270, sgl 100.0 ("value")) -> (w264:sgl)
                n238 = In Range and Coerce(upper limit=sgl 100.0, x=w264, lower limit=sgl 0.0 ("upper limit")) -> (coerced(x)=w261:sgl)  [unwired: 1 out]
              }
            }
            n239 = property on="Frequency [Hz]" class="DigNum (strict)"("Val(Sgnl)"=w247) -> ()  [unwired: 2 in, 2 out]
            n240 = property on="Duty Cycle [%]" class="DigNum (strict)"("Val(Sgnl)"=w246) -> ()  [unwired: 2 in, 2 out]
          }
          event "_AdaptMode": Value Change {
            n241 = event-data() -> ()  [unwired: 7 out]
            n242 = local read "_DiffIO Channels"() -> (w282:i32[])
            n243 = local read "AdaptMode"() -> (w290:u32)
            n244 = Number To Boolean Array(number=w290) -> (Boolean array=w284:bool[])
            n245 = for {
              shift-right: [w293] -> w283
              shift-left: w284 -> [w292]
              tunnel: w282 -> [w294] mode=indexing
              tunnel: "_AdaptMode" -> [w291]
              n246 = Replace Array Subset(array=w292, new element=w291, index=w294) -> (w293:bool[])
            }
            n247 = Boolean Array To Number(Boolean array=w283) -> (number=w289:u32)
            n248 = Select(t=T7."Disabled and Grayed Out" ("Disabled"), s="_AdaptMode", f=T7."Enabled" ("Disabled")) -> (s? t:f=w285:T7)
            n249 = property on="AdaptMode" class="DigNum (strict)"("Val(Sgnl)"=w289) -> ()  [unwired: 2 in, 2 out]
            n250 = property on="_SetupElement" class="Clust (strict)"("DisabledEnum"=w285) -> ()  [unwired: 2 in, 2 out]
            n251 = property on="_PWM Settings Element" class="Clust (strict)"("DisabledEnum"=w285, "Val(Sgnl)"=T6 {"PWM-TimingMode"=enum."Frequency", "PWM-Frequency"=0.0, "PWM-Period"=0.0, "PWM-ControlMode"=enum."Duty Cycle", "PWM-DutyCycle"=0.0, "PWM-PulseWidth"=0.0} ("Value (Signaling)")) -> ()  [unwired: 2 in, 2 out]
            n252 = property on="_Refresh" class="Bool (strict)"("Val(Sgnl)"=TRUE ("Value (Signaling)")) -> ()  [unwired: 2 in, 2 out]
          }
          event "_DiffIO Channels": Value Change {
            n253 = event-data() -> ()  [unwired: 2 out]
            n254 = property on="_Refresh" class="Bool (strict)"("Val(Sgnl)"=TRUE ("Value (Signaling)")) -> ()  [unwired: 2 in, 2 out]
          }
          event "_Refresh": Value Change {
            n255 = event-data() -> ()  [unwired: 2 out]
            n256 = local write "_Refresh"(FALSE ("_Refresh")) -> ()
            n257 = stacked-sequence {
              frame #0 {
                n258 = call <vilib>:"Set Busy.vi"() -> ()  [unwired: 10 in, 2 out]
                n259 = Wait (ms)(milliseconds to wait=u32 100) -> ()  [unwired: 1 out]
              }
              frame #1 {
                n260 = local read "_DiffIO Channels"() -> (w305:i32[])
                n261 = local read "ChannelNames"() -> (w313:string)
                n262 = local read "AdaptMode"() -> (w317:u32)
                n263 = local read "PWMSettings"() -> (w304:T5)
                n264 = local read "Filters"() -> (w302:sgl[])
                n265 = local read "Results"() -> (w299:T4[])
                n266 = local read "Setup"() -> (w320:T1[])
                n267 = Index Array(array=w305, index=0) -> (element=w298:i32)
                n268 = Spreadsheet String To Array(delimiter (Tab)=";", format string="%s", spreadsheet string=w313, array type (2D Dbl)=string[] []) -> (array=w311:string[])
                n269 = Number To Boolean Array(number=w317) -> (Boolean array=w316:bool[])
                n270 = Index Array(array=w320, index=w298) -> (element=w319:T1)
                n271 = Index Array(array=w299, index=w298) -> (element=w300:T4)
                n272 = Index Array(array=w304, index=w298) -> (element=w306:T6)
                n273 = Index Array(array=w311, index=w298) -> (element=w318:string)
                n274 = Index Array(array=w316, index=w298) -> (element=w308:bool)
                n275 = Index Array(array=w302, index=w298) -> (element=w301:sgl)
                n276 = local write "_AdaptMode"(w308) -> ()
                n277 = local write "_PWM Settings Element"(w306) -> ()
                n278 = local write "_SetupElement"(w319) -> ()
                n279 = local write "_ResultsElement"(w300) -> ()
                n280 = Select(t=T7."Disabled and Grayed Out" ("Disabled"), s=w308, f=T7."Enabled" ("Disabled")) -> (s? t:f=w307:T7)
                n281 = local write "_Filter"(w301) -> ()
                n282 = local write "_Channel Name"(w318) -> ()
                n283 = property on="_SetupElement" class="Clust (strict)"("DisabledEnum"=w307) -> ()  [unwired: 2 in, 2 out]
              }
              frame #2 {
                n284 = local read "ChannelNames"() -> (w332:string)
                n285 = Spreadsheet String To Array(delimiter (Tab)=";", format string="%s", spreadsheet string=w332, array type (2D Dbl)=string[] []) -> (array=w331:string[])
                n286 = control-ref of="_SetupElement"() -> (w326:refnum<vi>)
                n287 = control-ref of="_DiffIO Channels"() -> (w324:refnum<vi>)
                n288 = local read "_SetupElement"() -> (w321:T1)
                n289 = local read "_AdaptMode"() -> (w322:bool)
                n290 = local read "AdaptMode"() -> (w329:u32)
                n291 = local read "Results"() -> (w328:T4[])
                n292 = local read "Filters"() -> (w323:sgl[])
                n293 = local read "Setup"() -> (w335:T1[])
                n294 = control-ref of="_PWM Settings Element"() -> (w325:refnum<vi>)
                n295 = local read "State"() -> (w327:u8)
                n296 = call "DiffIO Command Disable.vi"("_Setup"=w326) -> ()  [unwired: 11 in]
                n297 = call "DiffIO PWM Disable.vi"("Adapting?"=w322, "_SetupElement"=w321, "Cluster in"=w325) -> ()  [unwired: 9 in]
                n298 = call "Refresh DiffIO Listbox.vi"("_DiffIOState"=w327, "AdaptMode"=w329, "Results"=w328, "DigitalFilter"=w323, "Command"=w335, "Names"=w331, "_DiffIO Channels"=w324) -> ()  [unwired: 5 in]
              }
              frame #3 {
                n299 = call <vilib>:"Unset Busy.vi"() -> ()  [unwired: 11 in, 1 out]
              }
            }
          }
        }
      }
    }
  }
